vi "getData.vi"(11 "DLRS1ADisplacementGauge in":refnum<class "DLRS1ADisplacementGauge.lvclass">) -> (2 "DLRS1ADisplacementGaugeData":T1, 3 "DLRS1ADisplacementGauge out":refnum<class "DLRS1ADisplacementGauge.lvclass">)   [LabVIEW 2016, in "RTDLRS1ADisplacementGauge.lvlib" / "DLRS1ADisplacementGauge.lvclass"]
uses:
  DLRS1ADisplacementGauge.lvclass
  DataTypes/DLRS1ADisplacementGaugeData.ctl
  DataTypes/DLRS1ADisplacementGaugeTelemetry.ctl
  DataTypes/DLRS1ADisplacementGaugeResponses.ctl
  DataTypes/DLRS1ADisplacementGaugeErrors.ctl
  DLRS1ADisplacementGauge.lvclass/DLRS1ADisplacementGauge.ctl
  RTDLRS1ADisplacementGauge.lvlib
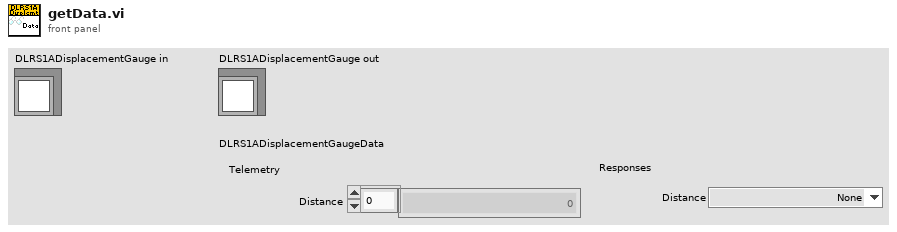
[diagram p1: front panel]
types:
  T1 = typedef "RTDLRS1ADisplacementGauge.lvlib/DLRS1ADisplacementGaugeData.ctl" = cluster{"Telemetry":T2, "Responses":T3}
  T2 = typedef "RTDLRS1ADisplacementGauge.lvlib/DLRS1ADisplacementGaugeTelemetry.ctl" = cluster{"Distance":dbl[]}
  T3 = typedef "RTDLRS1ADisplacementGauge.lvlib/DLRS1ADisplacementGaugeResponses.ctl" = cluster{"Distance":T4}
  T4 = typedef "RTDLRS1ADisplacementGauge.lvlib/DLRS1ADisplacementGaugeErrors.ctl" = enum8{"None", "InvalidCommand", "CommunicationTimeoutError", "DataLengthError", "NumberOfParametersError", "ParameterError", "CommunicationError", "IDNumberError", "ExpansionLineError", "WriteControlError", "UnknownError", "UnknownResponseError"}
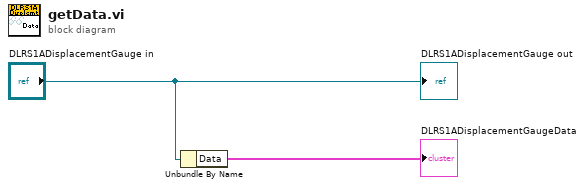
[diagram p0: block diagram]
diagram:
  n1 = Unbundle By Name("DLRS1ADisplacementGauge in") -> ("Data"=→"DLRS1ADisplacementGaugeData":T1)
  "DLRS1ADisplacementGauge out" <- "DLRS1ADisplacementGauge in"
